vi "PID current time.vi"() -> (8 "current time (sec)":dbl format="%.2f")   [LabVIEW 2016]
doc: "This one-shot VI returns the current time in seconds\n\nPaul K Dixon\nPhysics 350\nCSUSB Physics"
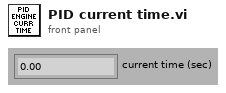
[diagram p1: front panel]
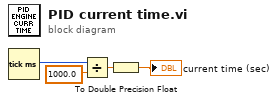
[diagram p0: block diagram]
diagram:
  n1 = Tick Count (ms)() -> (millisecond timer value=w3:u32)
  n2 = Divide(x=w3, y=1000.0) -> (x/y=w1:dbl)
  n3 = To Double Precision Float(number=w1) -> (double precision float=→"current time (sec)":dbl)
